vi "初始化.vi"(8 "error in (no error)":errorcluster caption="错误输入（无错误）", 10 "类私有数据的簇":T1, 11 "程序 输入":refnum<class "程序.lvclass">) -> (0 "error out":errorcluster caption="错误输出", 3 "程序 输出":refnum<class "程序.lvclass">)   [LabVIEW 2018, in "程序.lvclass"]
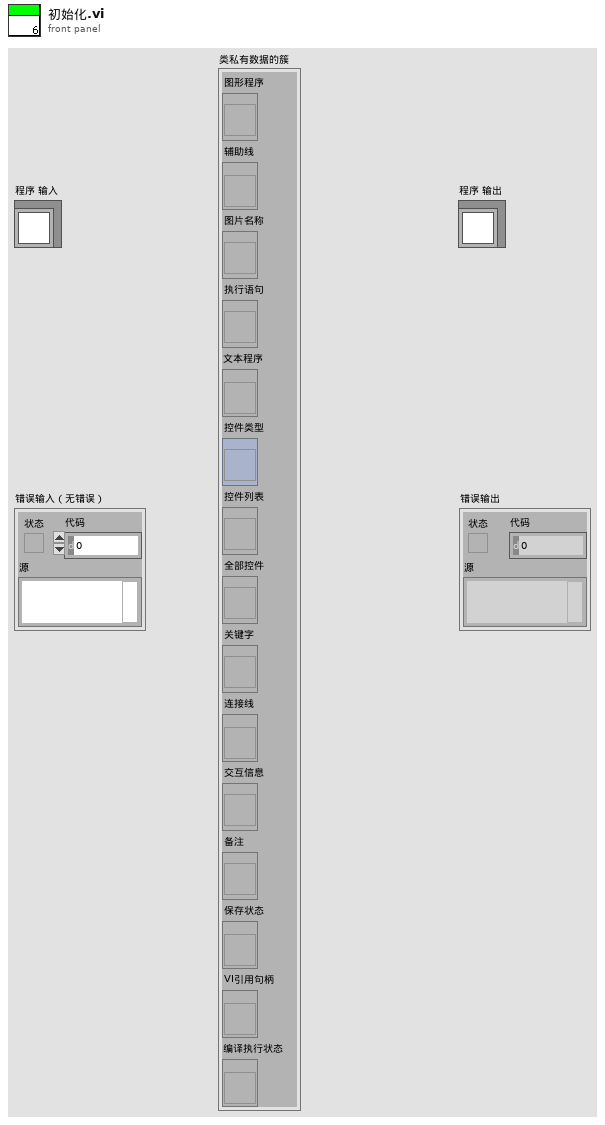
[diagram p1: front panel]
types:
  T1 = cluster{"图形程序":refnum<vi>, "辅助线":refnum<vi>, "图片名称":refnum<vi>, "执行语句":refnum<vi>, "文本程序":refnum<vi>, "控件类型":refnum<vi>, "控件列表":refnum<vi>, "全部控件":refnum<vi>, "关键字":refnum<vi>, "连接线":refnum<vi>, "交互信息":refnum<vi>, "备注":refnum<vi>, "保存状态":refnum<vi>, "VI引用句柄":refnum<vi>, "编译执行状态":refnum<vi>}
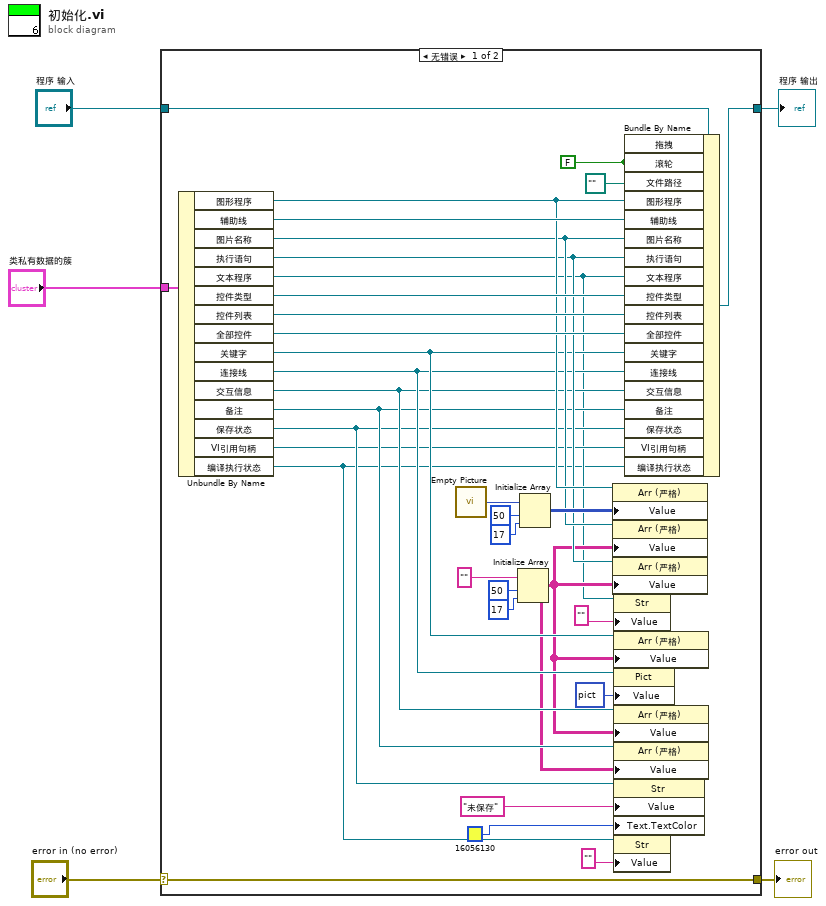
[diagram p0: block diagram]
diagram:
  n1 = case shown="无错误" "error in (no error)" {
    selector: "error in (no error)" -> [w39 w41]
    tunnel: [w39 w41] -> w4
    tunnel: [w37 w40] -> w2
    tunnel: "程序 输入" -> [w38 w40]
    tunnel: "类私有数据的簇" -> [w36 _]
    frame No Error {
      w9 = FALSE ("滚轮")
      n2 = Unbundle By Name(w36) -> ("图形程序"=w31:refnum<vi>, "辅助线"=w35:refnum<vi>, "图片名称"=w25:refnum<vi>, "执行语句"=w22:refnum<vi>, "文本程序"=w7:refnum<vi>, "控件类型"=w34:refnum<vi>, "控件列表"=w33:refnum<vi>, "全部控件"=w32:refnum<vi>, "关键字"=w20:refnum<vi>, "连接线"=w19:refnum<vi>, "交互信息"=w17:refnum<vi>, "备注"=w16:refnum<vi>, "保存状态"=w13:refnum<vi>, "VI引用句柄"=w10:refnum<vi>, "编译执行状态"=w6:refnum<vi>)
      n3 = call "Empty Picture"() -> ("empty picture"=w28:picture)
      n4 = Initialize Array("", 50 ("维数大小"), 17 ("维数大小")) -> (w15:string[][])
      n5 = Initialize Array(w28, 50 ("维数大小"), 17 ("维数大小")) -> (w27:picture[][])
      n6 = property class="Arr (严格)"(reference=w31, "Value"=w27) -> ()  [unwired: 1 in, 2 out]
      n7 = property class="Arr (严格)"(reference=w25, "Value"=w15) -> ()  [unwired: 1 in, 2 out]
      n8 = property class="Arr (严格)"(reference=w22, "Value"=w15) -> ()  [unwired: 1 in, 2 out]
      n9 = property class="Str"(reference=w7, "Value"="" ("值")) -> ()  [unwired: 1 in, 2 out]
      n10 = property class="Arr (严格)"(reference=w20, "Value"=w15) -> ()  [unwired: 1 in, 2 out]
      n11 = property class="Pict"(reference=w19, "Value"=picture data[5B] ("值")) -> ()  [unwired: 1 in, 2 out]
      n12 = property class="Arr (严格)"(reference=w17, "Value"=w15) -> ()  [unwired: 1 in, 2 out]
      n13 = property class="Arr (严格)"(reference=w16, "Value"=w15) -> ()  [unwired: 1 in, 2 out]
      n14 = property class="Str"(reference=w13, "Value"="未保存" ("值"), "Text.TextColor"=u32 16056130) -> ()  [unwired: 1 in, 2 out]
      n15 = property class="Str"(reference=w6, "Value"="" ("值")) -> ()  [unwired: 1 in, 2 out]
      n16 = Bundle By Name(cluster=w38, "拖拽"=w9, "滚轮"=w9, "文件路径"=path "", "图形程序"=w31, "辅助线"=w35, "图片名称"=w25, "执行语句"=w22, "文本程序"=w7, "控件类型"=w34, "控件列表"=w33, "全部控件"=w32, "关键字"=w20, "连接线"=w19, "交互信息"=w17, "备注"=w16, "保存状态"=w13, "VI引用句柄"=w10, "编译执行状态"=w6) -> (w37:refnum<class "程序.lvclass">)
    }
    frame Error {
    }
  }
  "error out" <- w4
  "程序 输出" <- w2
